vi "cont_sampling_prodcons.vi"() -> ()   [LabVIEW 2013]
uses:
  <vilib>/DAQmx/create/channels.llb/DAQmx Create Channel (AI-Voltage-Basic).vi
  <vilib>/DAQmx/configure/timing.llb/DAQmx Timing (Sample Clock).vi
  <vilib>/DAQmx/read.llb/DAQmx Read (Analog 2D DBL NChan NSamp).vi
  <vilib>/express/express arith-compare/Formula/XNode/ExpressFormulaBlockNode.xnode
panel:
  in  "Refresh in (s)":i8=1
  out "dt":dbl
  in  "Lock In":bool
  out "dLD_RMS":dbl=-0.0
  out "MLD Sim.LIA (mV/V)":dbl=nan
  out "MLD LIA (mV/V)":dbl=0.0123978
  out "Lockin_freq":dbl=9.4676
  out "MLD SA (mV/V)":dbl
  out "1f Peak (mv/V)":dbl
  out "DC Voltage (V)":dbl=1.0 format="%0.2f"
  out "Spectrum":cluster{"f0":dbl, "df":dbl, "magnitude":dbl[]}(graph)={"f0"=0.0, "df"=inf, "magnitude"=[]}
  in  "Second Harmonic":bool
  in  "Lock-in-Amplifier VISA":refnum<visa-resource-name>="GPIB0::3::INSTR"
  out "Waveform Graph":waveform(dbl)[](graph)=[{"t0"=timestamp(0 s since 1904-01-01), "dt"=1.0, "Y"=[]}, {"t0"=timestamp(0 s since 1904-01-01), "dt"=1.0, "Y"=[]}]
  in  "AC?":bool
  out "levelB":dbl format="%#_2g"
  out "levelA":dbl format="%#_3g"
  in  "V/div B":dbl(knob)=0.2 scale=10.0..0.01 scale format="%#_3g"
  in  "level B":dbl(slide) scale=-1.0..1.0 scale format="%#_3g"
  in  "level A":dbl(slide) scale=-1.0..1.0 scale format="%#_3g"
  in  "V/div A":dbl(knob)=0.2 scale=10.0..0.01 scale format="%#.3f"
  out "2f frequency (Hz)":dbl=-inf
  out "Oscilloscope":waveform(dbl)[](graph)=[{"t0"=timestamp(0 s since 1904-01-01), "dt"=0.001, "Y"=[]}, {"t0"=timestamp(0 s since 1904-01-01), "dt"=0.001, "Y"=[]}]
  in  "rate":dbl=1000.0 format="%0.2f"
  in  "samples per channel":i32=1000
  in  "Sensitivity":T1(ring)
  in  "Reference Signal":tag="Dev1/ai1"
  in  "LD Signal":tag="Dev1/ai0" caption="LD Channel"
  in  "stop":bool
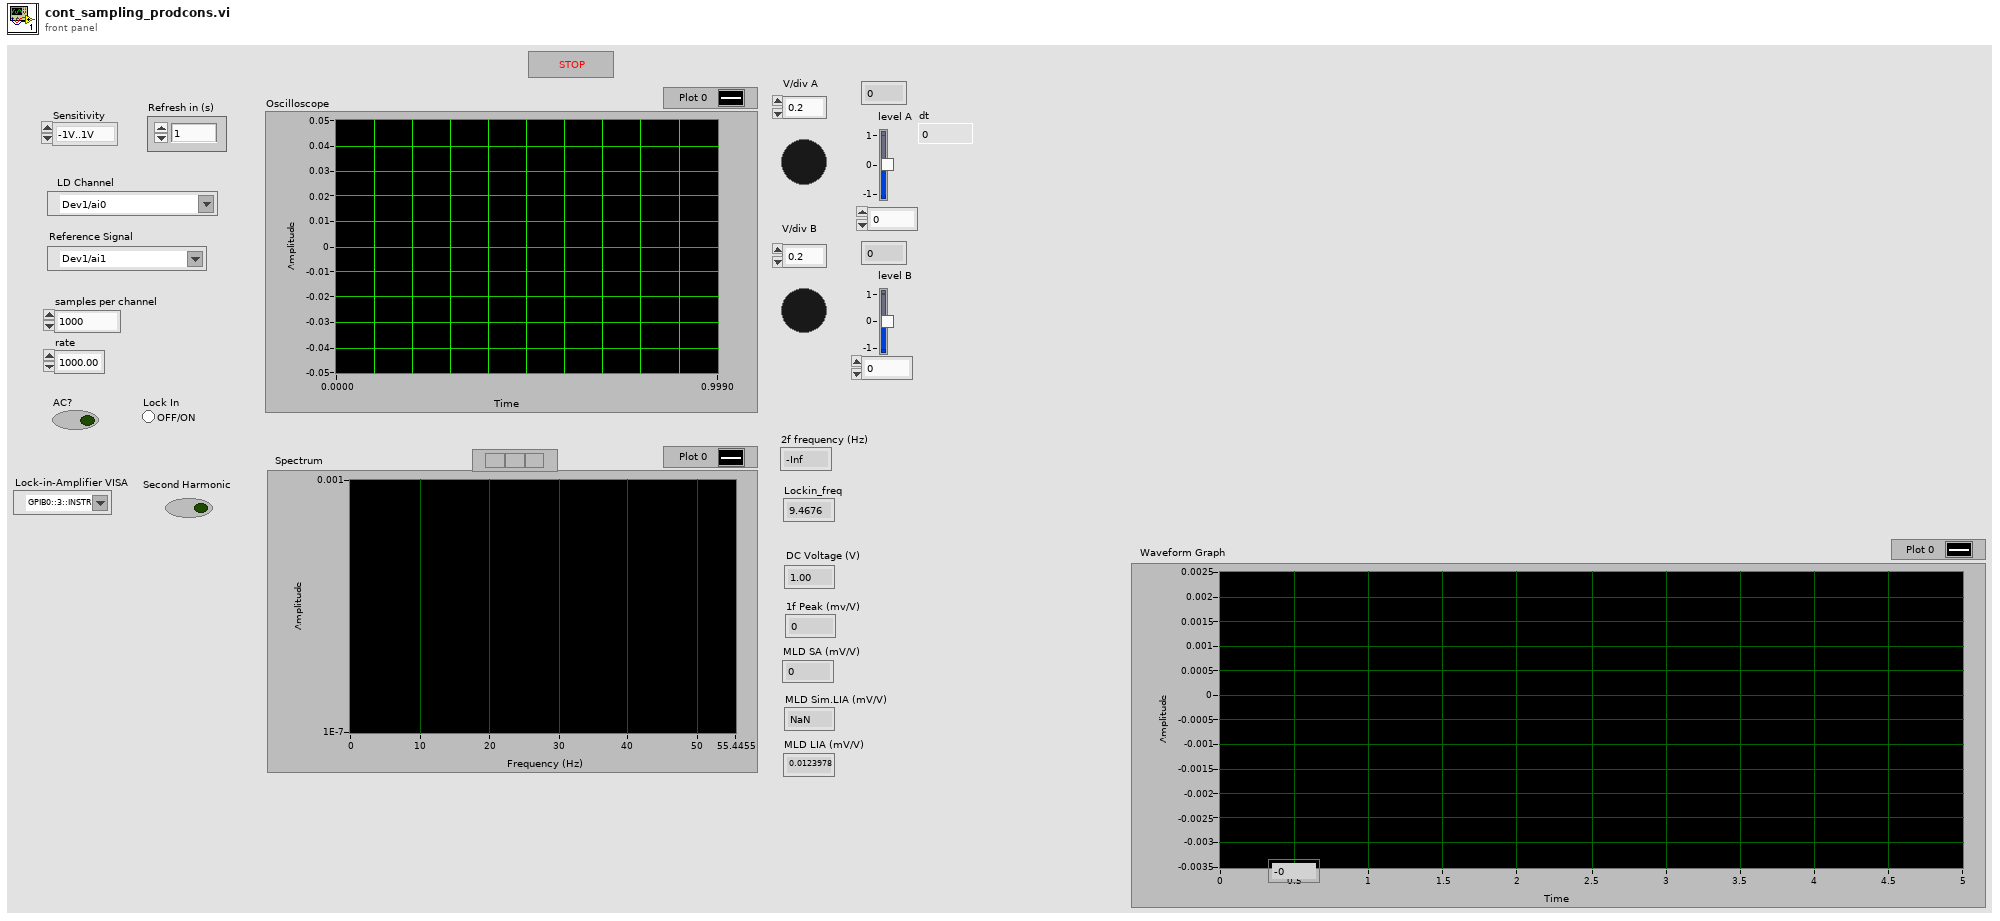
[diagram p1: front panel]
types:
  T1 = enum16{"-1V..1V", "-1.25V..1.25V", "-2V..2V", "-2.5V..2.5V", "-4V..4V", "-5V..5V", "-10V..10V"}
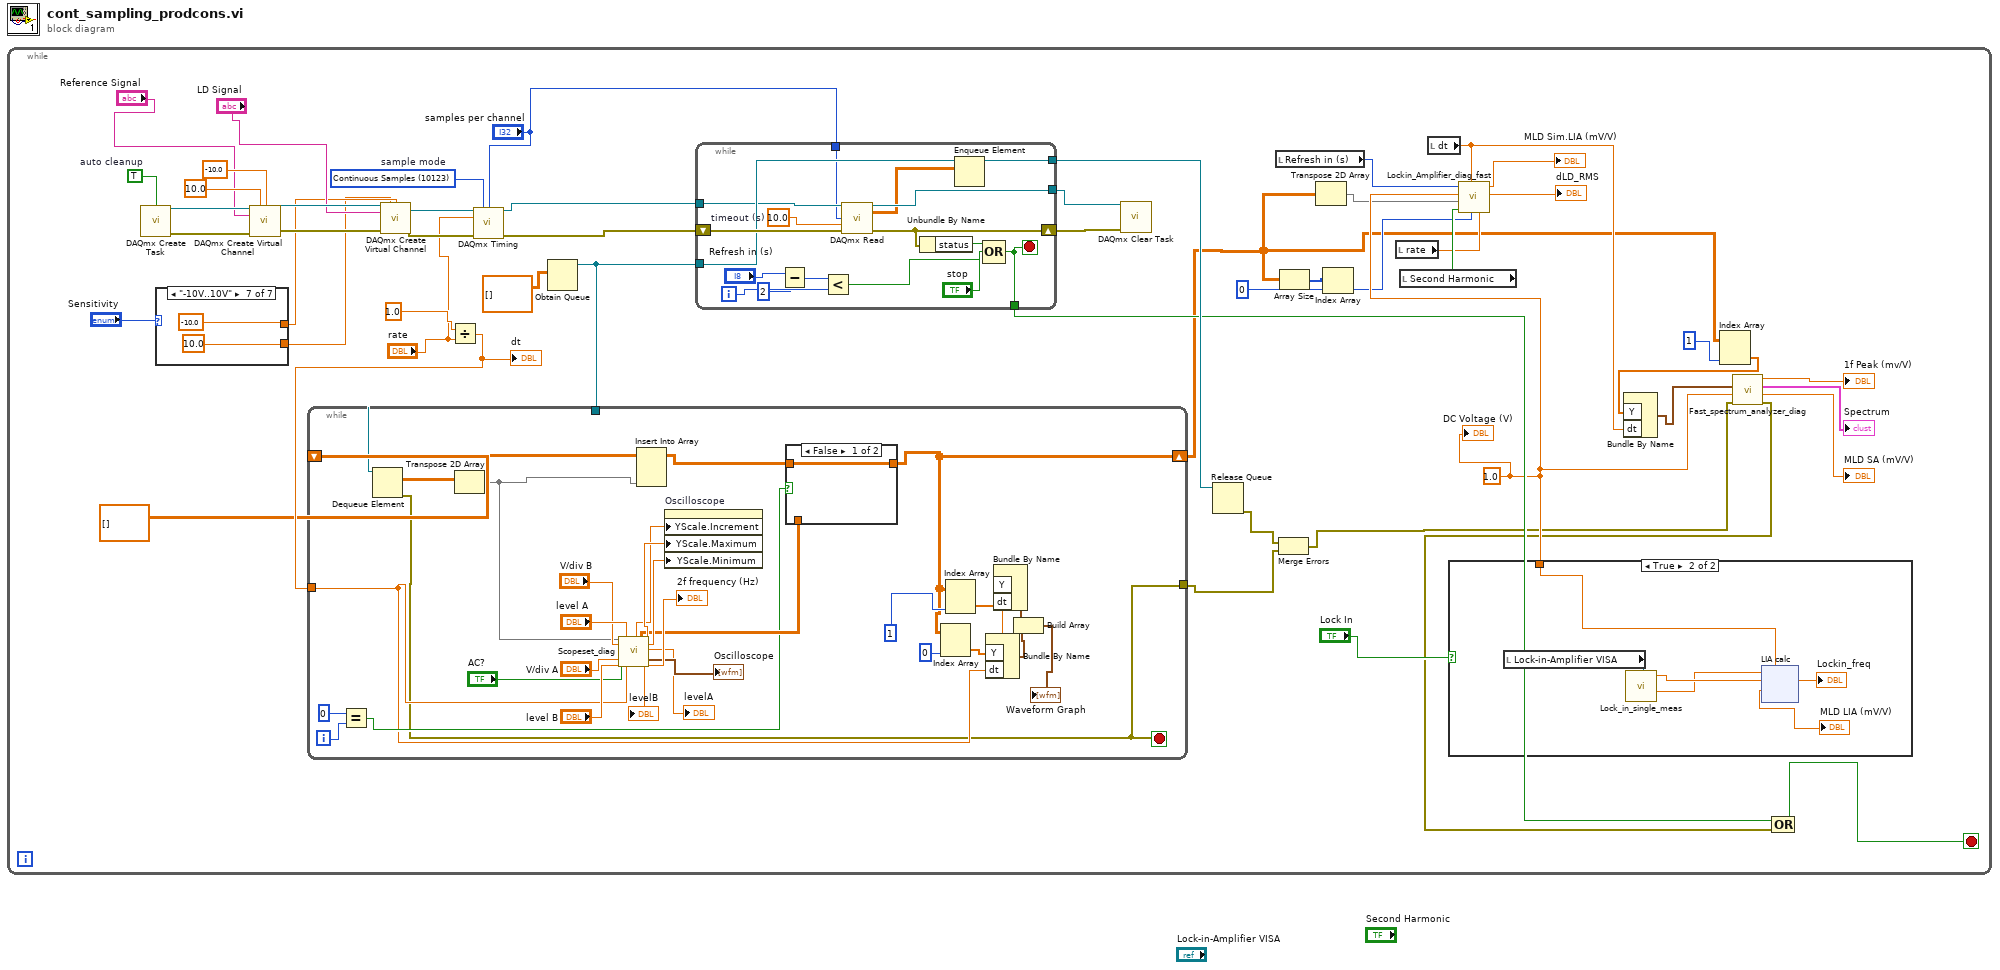
[diagram p0: block diagram]
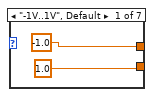
[diagram p3: hidden frame]
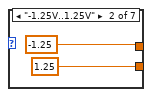
[diagram p4: hidden frame]
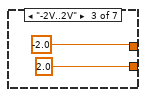
[diagram p5: hidden frame]
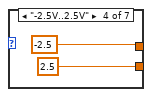
[diagram p6: hidden frame]
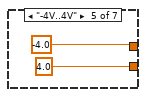
[diagram p7: hidden frame]
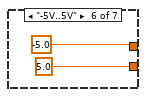
[diagram p8: hidden frame]
diagram:
  n1 = while {
    stop <- w13 stop-if-true
    w14 = 1.0 ("DC Voltage (V)")
    w45 = 10123 items=["Finite Samples"=10178, "Continuous Samples"=10123, "Hardware Timed Single Point"=12522]  # sample mode
    w37 = TRUE  # auto cleanup
    n2 = call <vilib>:"DAQmx Create Task.vi"("auto cleanup"=w37) -> ("task out"=w38:refnum<k21>, "error out"=w36:errorcluster)  [unwired: 13 in]
    n3 = case shown="\"-10V..10V\"" "Sensitivity" {
      tunnel: [-1.0 ("maximum value") -1.25 ("maximum value") -2.0 ("maximum value") -2.5 ("maximum value") -4.0 ("maximum value") -5.0 ("maximum value") -10.0 ("maximum value")] -> w32
      tunnel: [1.0 ("maximum value") 1.25 ("maximum value") 2.0 ("maximum value") 2.5 ("maximum value") 4.0 ("maximum value") 5.0 ("maximum value") 10.0 ("maximum value")] -> w31
      frame "-1V..1V", Default {
      }
      frame "-1.25V..1.25V" {
      }
      frame "-2V..2V" {
      }
      frame "-2.5V..2.5V" {
      }
      frame "-4V..4V" {
      }
      frame "-5V..5V" {
      }
      frame "-10V..10V" {
      }
    }
    n4 = call-poly <vilib>:"DAQmx Create Virtual Channel.vi"("task in"=w38, "maximum value"=10.0, "minimum value"=-10.0, "physical channels"="Reference Signal", "error in"=w36) -> ("task out"=w42:refnum<k21>, "error out"=w41:errorcluster)  [unwired: 9 in]
    n5 = call-poly <vilib>:"DAQmx Create Virtual Channel.vi"("task in"=w42, "maximum value"=w31, "minimum value"=w32, "physical channels"="LD Signal", "error in"=w41) -> ("task out"=w44:refnum<k21>, "error out"=w43:errorcluster)  [unwired: 9 in]
    n6 = Divide(x=1.0, y="rate") -> (x/y=w46:dbl)
    "dt" <- w46
    n7 = call-poly <vilib>:"DAQmx Timing.vi"("task/channels in"=w44, "sample mode"=w45, "samples per channel"="samples per channel", "rate"="rate", "error in"=w43) -> ("task out"=w30:refnum<k21>, "error out"=w29:errorcluster)  [unwired: 9 in]
    n8 = Obtain Queue(element data type=dbl[][] [] ("data")) -> (queue out=w50:refnum<queue>)  [unwired: 4 in, 2 out]
    n9 = while {
      tunnel: w50 -> [w112]
      tunnel: w46 -> [w83]
      shift-right: [w86] -> w2
      shift-left: dbl[][] [] ("element data type") -> [w95]
      tunnel: [w82] -> w4
      i -> [w98]
      stop <- w82 stop-if-true
      n10 = Equal?(x=0, y=w98) -> (x = y?=w92:bool)
      n11 = Dequeue Element(queue=w112) -> (element=w99:dbl[][], error out=w82:errorcluster)  [unwired: 2 in, 2 out]
      n12 = Transpose 2D Array(2D array=w99) -> (transposed array=w94:dbl[][])
      n13 = call "Scopeset_diag.vi"("Ref_MLD measurement"=w94, "V/div in B"="V/div B", "AC?"="AC?", "V/div in A"="V/div A", "level B"="level B", "level A"="level A", "dt"=w83) -> ("V/div out"=w106:dbl, "Ref_MLD_triggered"=w96:dbl[][], "levelB"=→"levelB":dbl, "Scale Max"=w108:dbl, "Scale Min"=w107:dbl, "levelA"=→"levelA":dbl, "Array"=→"Oscilloscope":waveform(dbl)[], "Frequency"=→"2f frequency (Hz)":dbl)  [unwired: 3 in, 2 out]
      n14 = Insert Into Array(array=w95, new element=w94) -> (w93:dbl[][])  [unwired: 2 in]
      n15 = property on="Oscilloscope" class="WFChart (strict)"("YScale.Increment"=w106, "YScale.Maximum"=w108, "YScale.Minimum"=w107) -> ()  [unwired: 2 in, 2 out]
      n16 = case shown="False" w92 {
        tunnel: w96 -> [_ w114]
        tunnel: w93 -> [w113 _]
        tunnel: [w113 w114] -> w86
        frame False {
        }
        frame True {
        }
      }
      n17 = Index Array(array=w86, index (col)=0 ("disabled index (col)")) -> (element=w84:dbl[])  [unwired: 1 in]
      n18 = Index Array(array=w86, index (col)=1 ("disabled index (col)")) -> (element=w85:dbl[])  [unwired: 1 in]
      n19 = Bundle By Name("Y"=w84, "dt"=w83) -> (w88:waveform(dbl))  [unwired: 1 in]
      n20 = Bundle By Name("Y"=w85, "dt"=w83) -> (w89:waveform(dbl))  [unwired: 1 in]
      n21 = Build Array(w89, w88) -> (→"Waveform Graph":waveform(dbl)[])
    }
    n22 = while {
      tunnel: [w130] -> w51
      shift-right: [w128] -> w52
      shift-left: w29 -> [w131]
      tunnel: [w125] -> w16
      tunnel: w50 -> [w124]
      tunnel: [w122] -> w49
      tunnel: w30 -> [w121]
      tunnel: "samples per channel" -> [w120]
      i -> [w119]
      stop <- w125 stop-if-true
      w126 = 10.0  # timeout (s)
      n23 = Subtract(x="Refresh in (s)", y=i8 2) -> (x-y=w117:i8)
      n24 = Less?(x=w117, y=w119) -> (x < y?=w118:bool)
      n25 = call-poly <vilib>:"DAQmx Read.vi"("task/channels in"=w121, "number of samples per channel"=w120, "timeout"=w126, "error in"=w131) -> ("task out"=w130:refnum<k21>, "data"=w123:dbl[][], "error out"=w128:errorcluster)  [unwired: 9 in]
      n26 = Unbundle By Name(w128) -> ("status"=w129:bool)
      n27 = Enqueue Element(queue=w124, element=w123) -> (queue out=w122:refnum<queue>)  [unwired: 2 in, 2 out]
      n28 = Compound Arithmetic op=OR(w129, "stop", w118) -> (w125:bool)
    }
    n29 = call <vilib>:"DAQmx Clear Task.vi"("task in"=w51, "error in"=w52) -> ()  [unwired: 13 in, 1 out]
    n30 = Release Queue(queue=w49) -> (error out=w5:errorcluster)  [unwired: 2 in, 2 out]
    n31 = local read "Refresh in (s)"() -> (w7:i8)
    n32 = Merge Errors(w5, w4) -> (w3:errorcluster)
    n33 = Array Size(array=w2) -> (size(s)=w10:i32[])
    n34 = Transpose 2D Array(2D array=w2) -> (transposed array=w1:dbl[][])
    n35 = Index Array(array=w10, index=0) -> (element=w8:i32)
    n36 = local read "rate"() -> (w11:dbl)
    n37 = local read "Second Harmonic"() -> (w17:bool)
    n38 = local read "dt"() -> (w6:dbl)
    n39 = case shown="True" "Lock In" {
      tunnel: w14 -> [_ w53]
      frame False {
      }
      frame True {
        n40 = local read "Lock-in-Amplifier VISA"() -> (w57:refnum<visa-resource-name>)
        n41 = call "Lock_in_single_meas.vi"("Lock-in-Amplifier VISA"=w57) -> ("Lockin_ampl"=w55:dbl, "Freq"=→"Lockin_freq":dbl)  [unwired: 7 in, 2 out]
        n42 = xnode "LIA calc"("X1"=w55, "X2"=w53) -> ("Result"=→"MLD LIA (mV/V)":dbl)  [unwired: 1 in, 1 out]
      }
    }
    n43 = call "Lockin_Amplifier_diag_fast.vi"("Sampling frequency"=w11, "Number of samples"=w8, "dt"=w6, "Second"=w17, "Ref_MLD measurement"=w1, "mean"=w14, "Refresh in (s)"=w7) -> ("Result"=→"dLD_RMS":dbl, "Result 2"=→"MLD Sim.LIA (mV/V)":dbl)  [unwired: 3 in]
    n44 = Index Array(array=w2, index (col)=1 ("disabled index (col)")) -> (element=w18:dbl[])  [unwired: 1 in]
    n45 = Bundle By Name("Y"=w18, "dt"=w6) -> (w20:waveform(dbl))  [unwired: 1 in]
    n46 = call "Fast_spectrum_analyzer_diag.vi"("error in (no error)"=w3, "mean"=w14, "Waveform"=w20) -> ("error out"=w12:errorcluster, "MLD SA (mV/V)"=→"MLD SA (mV/V)":dbl, "Spectrum (mV/V)"=→"Spectrum":cluster{"f0":dbl, "df":dbl, "magnitude":dbl[]}, "1f Peak (mv/V)"=→"1f Peak (mv/V)":dbl)  [unwired: 5 in]
    n47 = Compound Arithmetic op=OR(w16, w12) -> (w13:bool)
    "DC Voltage (V)" <- w14
  }
